vi "Configure Timer Trigger.vi"(0 "VISA resource name":refnum<visa-resource-name>, 1 "Start Time (in Sec)":dbl=1e-05, 5 "Timer Number (1)":u32=1 min=1 max=4 step=1, 7 "Count":i32=1 min=0 max=1048575 step=1, 9 "Delay":dbl=1e-05, 11 "error in (no error)":errorcluster, 12 "Start Time (fractional)":dbl=1e-05, 13 "Stimulus Event":u16(ring) items=["None", "Front Pannel Trigger Key", "Notify Trigger Block 1", "Notify Trigger Block 2", "Notify Trigger Block 3", "Notify Trigger Block 4", "Notify Trigger Block 5", "Notify Trigger Block 6", "Notify Trigger Block 7", "Notify Trigger Block 8", "Command", "Digi IO Line 1", "Digi IO Line 2", "Digi IO Line 3", "Digi IO Line 4", "Digi IO Line 5", "Digi IO Line 6", "TSP-Link 1", "TSP-Link 2", "TSP-Link 3", "LAN 1", "LAN 2", "LAN 3", "LAN 4", "LAN 5", "LAN 6", "LAN 7", "LAN 8", "Blender 1", "Blender 2", "Timer 1", "Timer 2", "Timer 3", "Timer 4", "Analog Trigger", "External Trigger"]) -> (4 "VISA resource name out":refnum<visa-resource-name>, 15 "error out":errorcluster)   [LabVIEW 2017, in "Keithley DMM7510.lvlib"]
doc: "This VI sets the logic on which the trigger event detector and the output trigger generator operate on the given trigger line. Also sets the IP address, protocol type ans stimulus event."
uses:
  Keithley DMM7510.lvlib
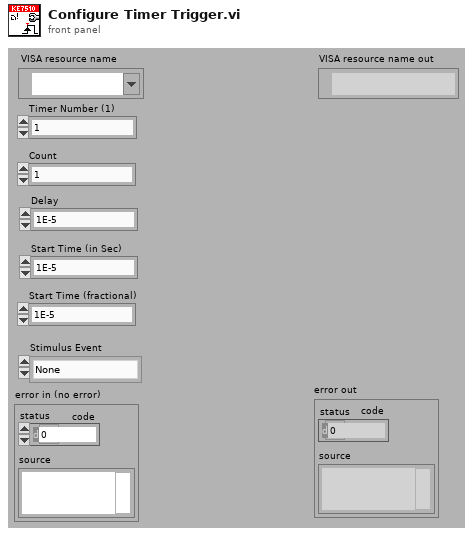
[diagram p1: front panel]
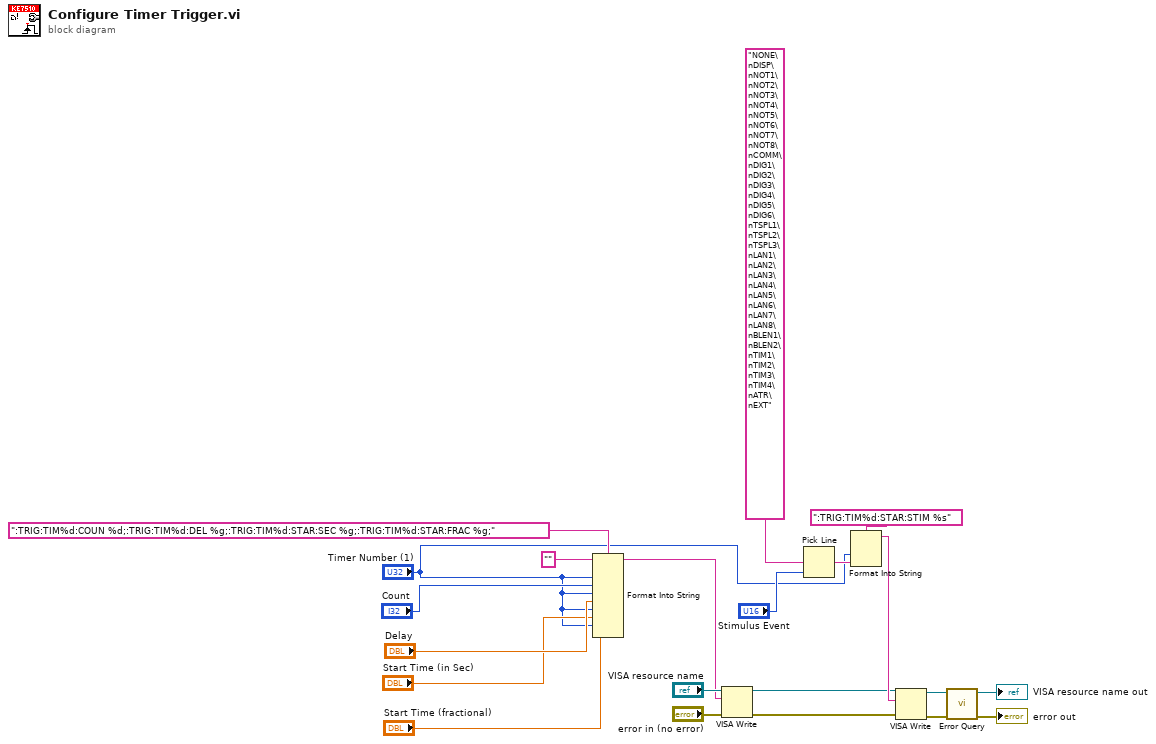
[diagram p0: block diagram]
diagram:
  n1 = Format Into String(format string=":TRIG:TIM%d:COUN %d;:TRIG:TIM%d:DEL %g;:TRIG:TIM%d:STAR:SEC %g;:TRIG:TIM%d:STAR:FRAC %g;", initial string="", "Timer Number (1)", "Count", "Timer Number (1)", "Delay", "Timer Number (1)", "Start Time (in Sec)", "Timer Number (1)", "Start Time (fractional)") -> (resulting string=w15:string)  [unwired: 1 in, 1 out]
  n2 = VISA Write(VISA resource name="VISA resource name", write buffer=w15, error in (no error)="error in (no error)") -> (VISA resource name out=w7:refnum<visa-resource-name>, error out=w6:errorcluster)  [unwired: 1 out]
  n3 = Pick Line(multi-line string="NONE\nDISP\nNOT1\nNOT2\nNOT3\nNOT4\nNOT5\nNOT6\nNOT7\nNOT8\nCOMM\nDIG1\nDIG2\nDIG3\nDIG4\nDIG5\nDIG6\nTSPL1\nTSPL2\nTSPL3\nLAN1\nLAN2\nLAN3\nLAN4\nLAN5\nLAN6\nLAN7\nLAN8\nBLEN1\nBLEN2\nTIM1\nTIM2\nTIM3\nTIM4\nATR\nEXT", line index="Stimulus Event") -> (output string=w12:string)  [unwired: 1 in]
  n4 = Format Into String(format string=":TRIG:TIM%d:STAR:STIM %s", "Timer Number (1)", w12) -> (resulting string=w8:string)  [unwired: 2 in, 1 out]
  n5 = VISA Write(VISA resource name=w7, write buffer=w8, error in (no error)=w6) -> (VISA resource name out=w9:refnum<visa-resource-name>, error out=w10:errorcluster)  [unwired: 1 out]
  n6 = call "Error Query.vi"("error in (no error)"=w10, "VISA resource name"=w9) -> ("error out"=→"error out":errorcluster, "VISA resource name out"=→"VISA resource name out":refnum<visa-resource-name>)  [unwired: 8 out]
